vi "temptest.vi"() -> ()   [LabVIEW 2010]
panel:
  in  "Numeric 3":dbl
  in  "mode (0) 2":i16
  in  "mode (0)":i16
  in  "Numeric 2":dbl
  out "Numeric":dbl
  out "error out 2":errorcluster
  out "XY Graph":cluster{dbl[], dbl[]}(graph)
  in  "Wait/s":dbl format="%.2f"
  in  "Step":dbl format="%.2f"
  in  "error in (no error)":errorcluster
  in  "Stop":dbl format="%.2f"
  in  "Start":dbl format="%.2f"
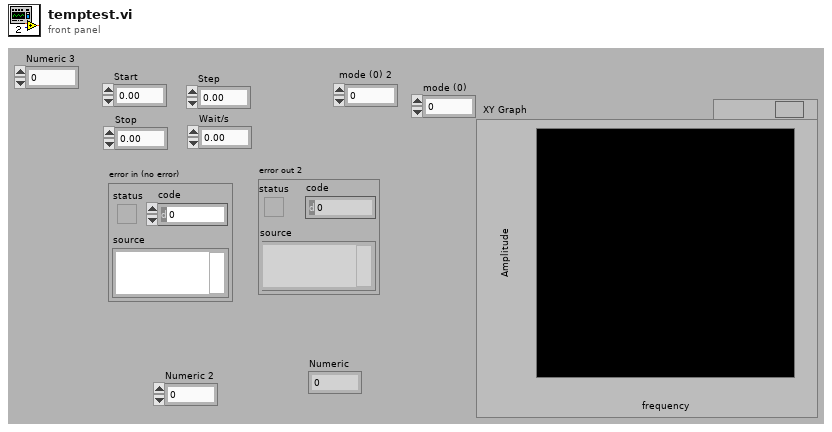
[diagram p1: front panel]
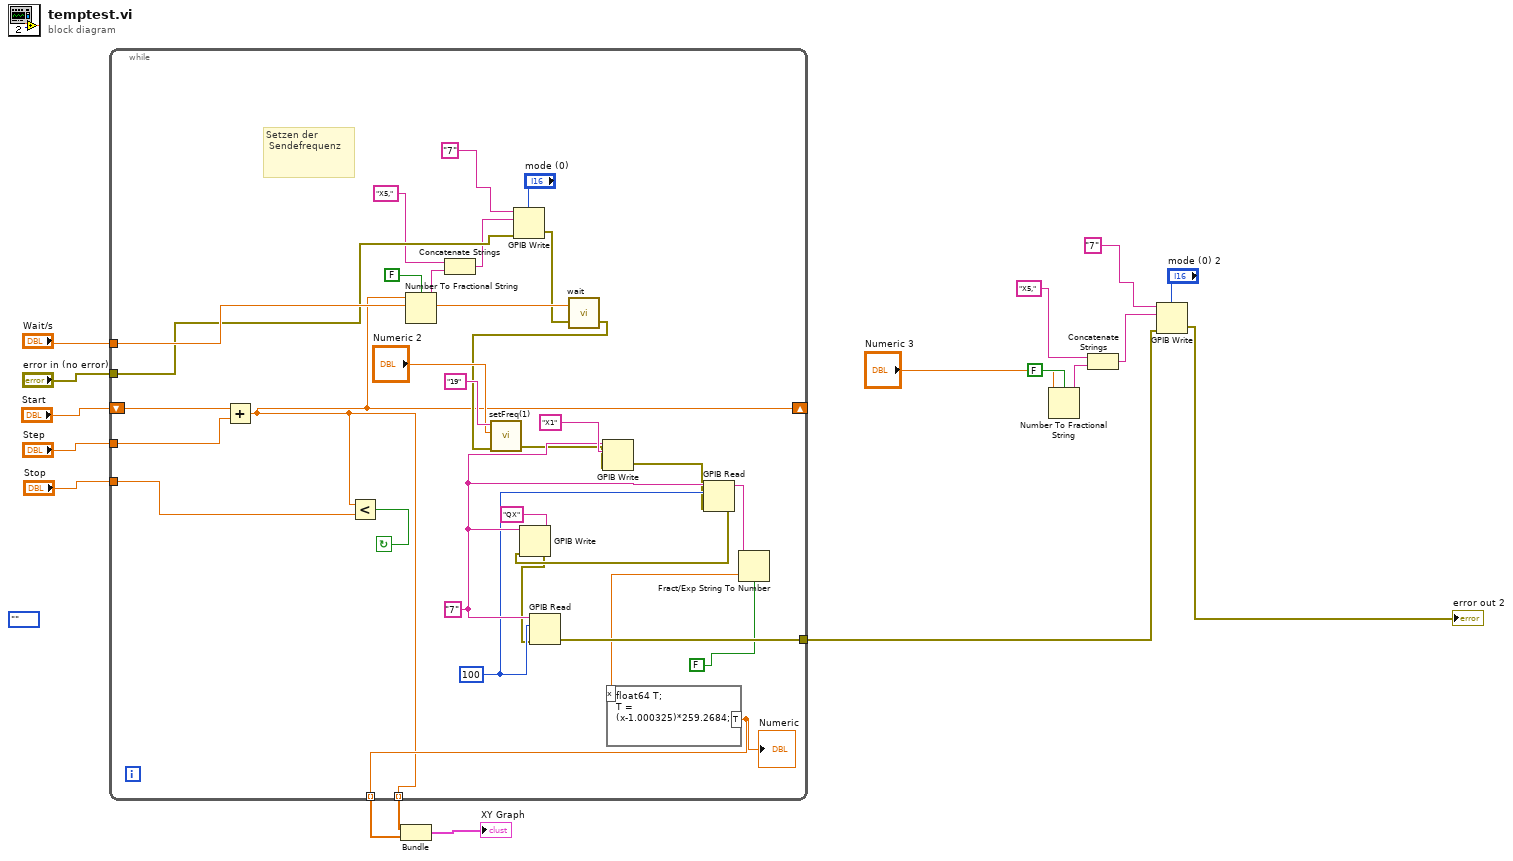
[diagram p0: block diagram]
diagram:
  (unwired) enum16{""}.""
  n1 = while {
    tunnel: "error in (no error)" -> [w21]
    shift-right: [w22] -> _
    shift-left: "Start" -> [w45]
    tunnel: "Step" -> [w47]
    tunnel: "Stop" -> [w46]
    tunnel: "Wait/s" -> [w43]
    tunnel: [w41] -> w2
    tunnel: [w25] -> w11 mode=indexing
    tunnel: [w22] -> w10 mode=indexing
    stop <- w44 continue-if-true
    w36 = 100
    w38 = "7"
    # "Setzen der \n Sendefrequenz"
    n2 = Add(x=w45, y=w47) -> (x+y=w22:dbl)
    n3 = Less?(x=w22, y=w46) -> (x < y?=w44:bool)
    n4 = Number To Fractional String(use system decimal point (T)=FALSE, number=w22) -> (F-format string=w20:string)  [unwired: 2 in]
    n5 = Concatenate Strings("X5,", w20) -> (w18:string)
    n6 = GPIB Write(0:"7", 1:w18, 2:"mode (0)", 3:w21) -> (6:w24:errorcluster)  [unwired: 1 in, 1 out]
    n7 = call "wait.vi"("error in"=w24, "Wartezeit in Sek"=w43) -> ("error out"=w23:errorcluster)  [unwired: 1 in]
    n8 = call "setFreq(1).vi"("error in"=w23, "Frequenz in Hz"="Numeric 2", "address string"="19") -> ("error out"=w32:errorcluster)  [unwired: 3 in]
    n9 = GPIB Write(0:w38, 1:"X1", 3:w32) -> (6:w35:errorcluster)  [unwired: 2 in, 1 out]
    n10 = GPIB Read(0:w38, 1:w36, 3:w35) -> (5:w33:string, 7:w31:errorcluster)  [unwired: 2 in, 1 out]
    n11 = GPIB Write(0:w38, 1:"QX", 3:w31) -> (6:w30:errorcluster)  [unwired: 2 in, 1 out]
    n12 = GPIB Read(0:w38, 1:w36, 3:w30) -> (7:w41:errorcluster)  [unwired: 2 in, 2 out]
    n13 = Fract/Exp String To Number(use system decimal point (T)=FALSE, string=w33) -> (number=w34:dbl)  [unwired: 2 in, 1 out]
    n14 = formula code="float64 T;\nT = (x-1.000325)*259.2684;"("x"=w34) -> ("T"=w25:dbl)
    "Numeric" <- w25
  }
  n15 = Bundle(w10, w11) -> (→"XY Graph":cluster{dbl[], dbl[]})  [unwired: 1 in]
  n16 = Number To Fractional String(use system decimal point (T)=FALSE, number="Numeric 3") -> (F-format string=w6:string)  [unwired: 2 in]
  n17 = Concatenate Strings("X5,", w6) -> (w4:string)
  n18 = GPIB Write(0:"7", 1:w4, 2:"mode (0) 2", 3:w2) -> (6:→"error out 2":errorcluster)  [unwired: 1 in, 1 out]
